vi "Load Default Sequence.vi"(8 "error in":errorcluster, 9 "Select Sequence to Load":T1(ring), 10 "TestStand Engine":refnum<k7>, 11 "Application Manager":refnum<k7>) -> (0 "error out":errorcluster, 1 "Loaded?":bool, 2 "dup TestStand Engine":refnum<k7>, 3 "dup Application Manager":refnum<k7>)   [LabVIEW 2010]
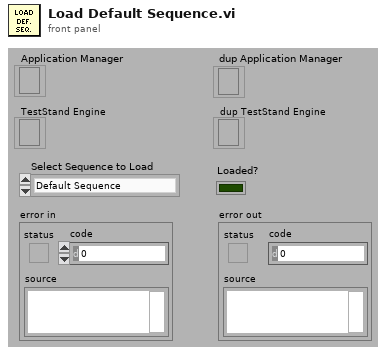
[diagram p1: front panel]
types:
  T1 = enum16{"Default Sequence", "Board Test Sequence"}
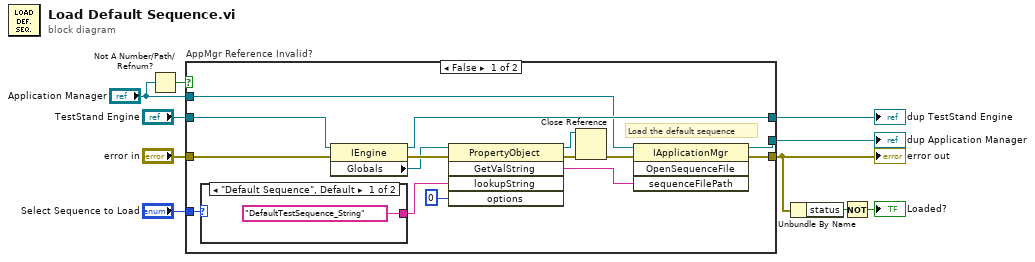
[diagram p0: block diagram]
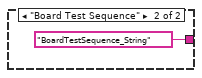
[diagram p2: hidden frame]
diagram:
  n1 = Not A Number/Path/Refnum?(number/path/refnum="Application Manager") -> (NaN/Path/Refnum?=w6:bool)
  n2 = case "AppMgr Reference Invalid?" shown="False" w6 {
    tunnel: [w25 w28] -> w10
    tunnel: "Application Manager" -> [w11 w28]
    tunnel: [w24 w29] -> w2
    tunnel: "TestStand Engine" -> [w22 w30]
    tunnel: "Select Sequence to Load" -> [w23 _]
    tunnel: "error in" -> [w13 w29]
    tunnel: [w12 w30] -> w4
    frame False {
      # "Load the default sequence"
      n3 = case shown="\"Default Sequence\", Default" w23 {
        tunnel: ["DefaultTestSequence_String" ("Lookup String") "BoardTestSequence_String" ("Lookup String")] -> w20
        frame "Default Sequence", Default {
        }
        frame "Board Test Sequence" {
        }
      }
      n4 = property class="IEngine"(reference=w22, error in=w13) -> (reference out=w12:refnum<k7>, error out=w21:errorcluster, "Globals"=w18:refnum<k7>)
      n5 = invoke class="PropertyObject" method="GetValString"(reference=w18, error in=w21, "lookupString"=w20, "options"=0) -> (reference out=w14:refnum<k7>, error out=w16:errorcluster, "GetValString"=w17:string)  [unwired: 1 in, 2 out]
      n6 = Close Reference(reference=w14, error in (no error)=w16) -> (error out=w15:errorcluster)
      n7 = invoke class="IApplicationMgr" method="OpenSequenceFile"(reference=w11, error in=w15, "sequenceFilePath"=w17) -> (reference out=w25:refnum<k7>, error out=w24:errorcluster)  [unwired: 1 in, 2 out]
    }
    frame True {
    }
  }
  "dup Application Manager" <- w10
  "error out" <- w2
  "dup TestStand Engine" <- w4
  n8 = Unbundle By Name(w2) -> ("status"=w3:bool)
  n9 = Not(x=w3) -> (.not. x?=→"Loaded?":bool)
